vi "getCalibPoint.vi"(9 "y size":i32, 10 "pixel angel (y)":dbl[](array[numeric]), 11 "Momentum [MeV/C]":dbl[](array[numeric])) -> (0 "Array":dbl[][](array[numeric]), 1 "XY Graph 2":cluster{"X":dbl, "Y":dbl}[](graph), 2 "Reference Points":T1, 3 "output cluster":T1, 4 "XY Graph":cluster{"X":dbl, "Y":dbl}[](graph))   [LabVIEW 2011]
uses:
  <vilib>/vision/Calibration.llb/Calibration Reference Points.ctl
  <vilib>/Analysis/1siggen.llb/Ramp Pattern by Delta.vi
  <vilib>/Analysis/NI_AALBase.lvlib
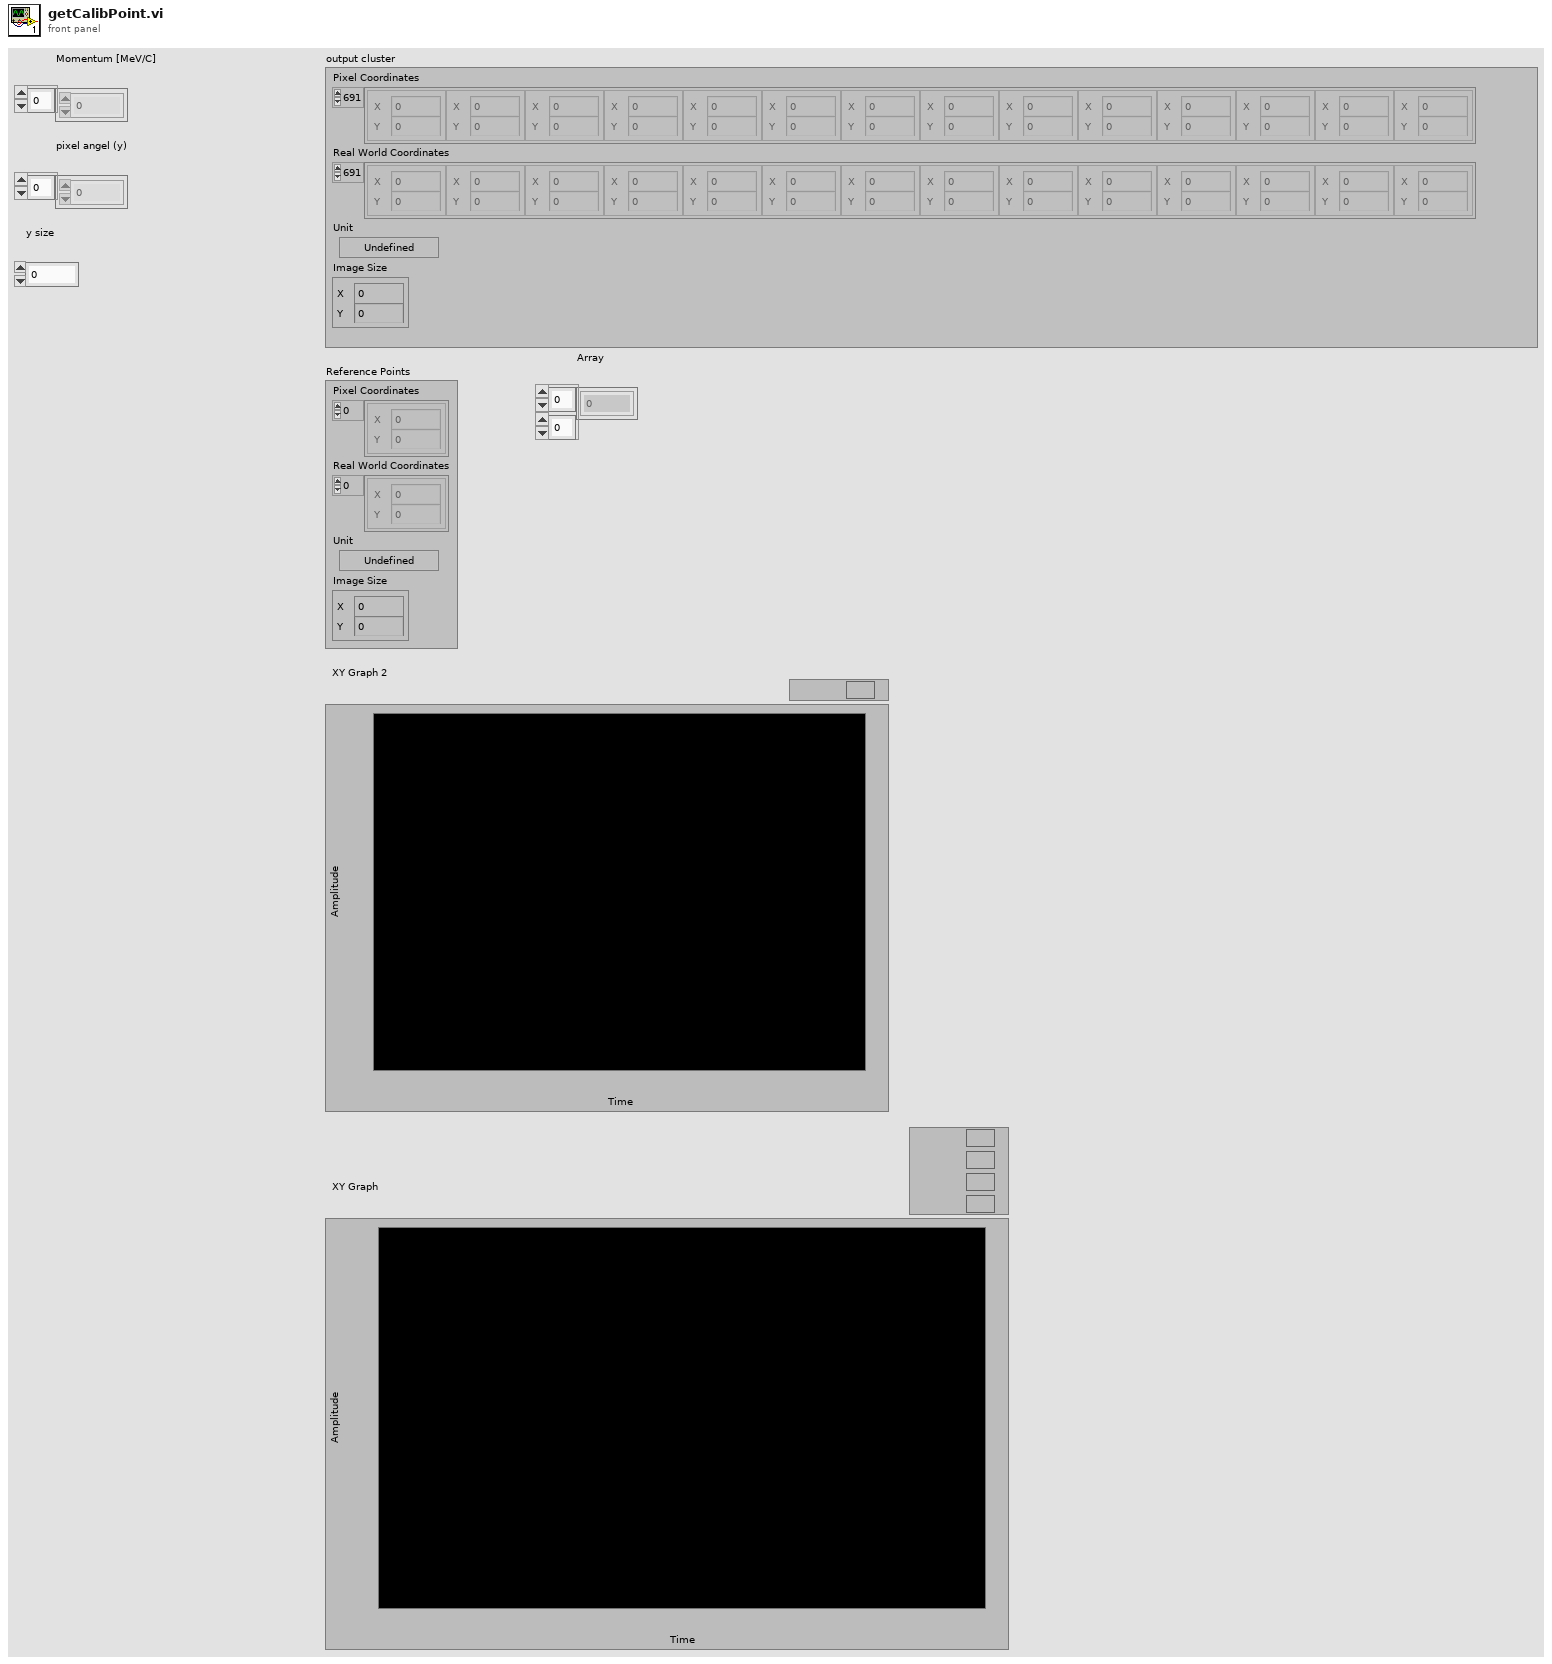
[diagram p1: front panel]
types:
  T1 = typedef "Calibration Reference Points.ctl" = cluster{"Pixel Coordinates":cluster{"X":dbl, "Y":dbl}[], "Real World Coordinates":cluster{"X":dbl, "Y":dbl}[], "Unit":T2, "Image Size":cluster{"X":u32, "Y":u32}}
  T2 = typedef "Image Unit" = enum32{"Undefined", "Angström", "Micrometer", "Millimeter", "Centimeter", "Meter", "Kilometer", "Microinch", "Inch", "Feet", "Nautical miles", "Standard miles", "Steps"}
  T3 = cluster{"Real Matrix Element":dbl, "Real Matrix Element":dbl}[]
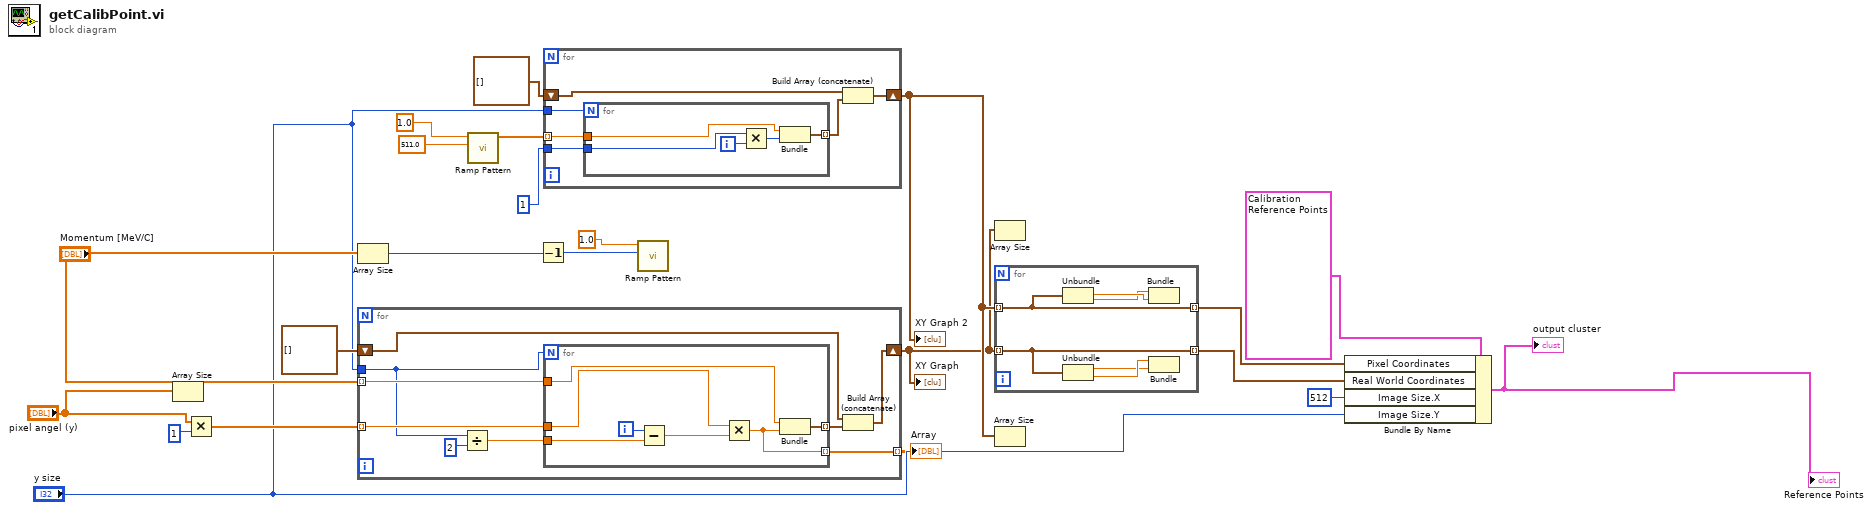
[diagram p0: block diagram]
diagram:
  n1 = Array Size(array="pixel angel (y)") -> ()  [unwired: 1 out]
  n2 = Multiply(x="pixel angel (y)", y=1) -> (x*y=w19:dbl[])
  n3 = Array Size(array="Momentum [MeV/C]") -> (size(s)=w10:i32)
  n4 = for {
    tunnel: "Momentum [MeV/C]" -> [w31] mode=indexing
    tunnel: "y size" -> [w26]
    shift-right: [w28] -> w20
    shift-left: cluster{dbl, dbl}[] [] -> [w29]
    tunnel: w19 -> [w27] mode=indexing
    tunnel: [w23] -> w1 mode=indexing
    n5 = Divide(x=w26, y=2) -> (x/y=w24:dbl)
    n6 = for {
      N: w26 -> [_]
      tunnel: w27 -> [w36]
      tunnel: w31 -> [w38]
      tunnel: [w37] -> w30 mode=indexing
      tunnel: w24 -> [w35]
      tunnel: [w32] -> w23 mode=indexing
      i -> [w33]
      n7 = Subtract(x=w33, y=w35) -> (x-y=w34:dbl)
      n8 = Multiply(x=w36, y=w34) -> (x*y=w32:dbl)
      n9 = Bundle(w38, w32) -> (w37:cluster{dbl, dbl})  [unwired: 1 in]
    }
    n10 = Build Array (concatenate)(w29, w30) -> (w28:cluster{dbl, dbl}[])
  }
  "XY Graph" <- w20
  "Array" <- w1
  n11 = call-poly <vilib>:"Ramp Pattern.vi"("end"=511.0, "delta"=1.0) -> ("Ramp Pattern"=w15:dbl[])  [unwired: 7 in, 2 out]
  n12 = Decrement(x=w10) -> (x-1=w11:i32)
  n13 = for {
    tunnel: w15 -> [w44] mode=indexing
    shift-right: [w42] -> w21
    shift-left: T3 [] -> [w41]
    tunnel: "y size" -> [w40]
    tunnel: 1 -> [w39]
    n14 = for {
      N: w40 -> [_]
      tunnel: w44 -> [w49]
      tunnel: [w48] -> w43 mode=indexing
      tunnel: w39 -> [w47]
      i -> [w45]
      n15 = Multiply(x=w47, y=w45) -> (x*y=w46:i32)
      n16 = Bundle(w49, w46) -> (w48:cluster{dbl, i32})  [unwired: 1 in]
    }
    n17 = Build Array (concatenate)(w41, w43) -> (w42:T3)
  }
  "XY Graph 2" <- w21
  n18 = call-poly <vilib>:"Ramp Pattern.vi"("end"=w11, "delta"=1.0) -> ()  [unwired: 7 in, 3 out]
  n19 = Array Size(array=w20) -> ()  [unwired: 1 out]
  n20 = for {
    tunnel: w21 -> [w50] mode=indexing
    tunnel: [w50] -> w7 mode=indexing
    tunnel: w20 -> [w51] mode=indexing
    tunnel: [w51] -> w8 mode=indexing
    n21 = Unbundle(w50) -> ("Real Matrix Element"=w55:dbl, "Real Matrix Element"=w54:dbl)
    n22 = Unbundle(w51) -> (w52:dbl, w53:dbl)
    n23 = Bundle("Real Matrix Element"=w54, "Real Matrix Element"=w55) -> ()  [unwired: 1 in, 1 out]
    n24 = Bundle(w53, w52) -> ()  [unwired: 1 in, 1 out]
  }
  n25 = Array Size(array=w21) -> ()  [unwired: 1 out]
  n26 = Bundle By Name(cluster=T1 {"Pixel Coordinates"=[{"X"=570.6379853095488, "Y"=340.45645330535154}, {"X"=647.5556818181818, "Y"=339.9465909090909}, {"X"=489.14118792599805, "Y"=340.794547224927}, {"X"=570.559915164369, "Y"=428.96182396606577}, {"X"=571.1038421599169, "Y"=251.64797507788163}, {"X"=719.6135802469136, "Y"=339.39012345679015}, {"X"=647.359212050985, "Y"=425.63731170336035}, {"X"=647.927355278093, "Y"=253.88081725312145}, {"X"=403.34514078110806, "Y"=341.1798365122616}, {"X"=489.36614173228344, "Y"=432.1003937007874}, {"X"=489.63300970873786, "Y"=249.25242718446603}, {"X"=570.873775843308, "Y"=516.2143634385201}, {"X"=571.809968847352, "Y"=163.4288681204569}, {"X"=786.8324396782842, "Y"=338.73458445040217}, {"X"=719.1072319201995, "Y"=422.27431421446386}, {"X"=719.8995098039215, "Y"=256.234068627451}, {"X"=647.1241134751773, "Y"=510.1111111111111}, {"X"=648.2274774774775, "Y"=168.53603603603602}, {"X"=313.9448751076658, "Y"=341.3255813953488}, {"X"=403.84508348794066, "Y"=434.9007421150278}, {"X"=404.0036199095023, "Y"=247.020814479638}, {"X"=490.1742654508612, "Y"=521.9088145896657}, {"X"=490.8612997090204, "Y"=158.447138700291}, {"X"=571.4618834080718, "Y"=601.1838565022422}, {"X"=572.9046121593292, "Y"=76.90041928721175}, {"X"=849.2731277533039, "Y"=338.05286343612335}, {"X"=786.2282608695652, "Y"=418.85733695652175}, {"X"=787.0280748663101, "Y"=258.451871657754}, {"X"=718.5839694656488, "Y"=504.147582697201}, {"X"=720.0232843137255, "Y"=173.4950980392157}, {"X"=647.0180940892642, "Y"=592.6731001206273}, {"X"=648.7929465301479, "Y"=84.46416382252559}, {"X"=221.77860082304528, "Y"=341.1670781893004}, {"X"=314.82819383259914, "Y"=437.3339207048458}, {"X"=314.7304721030043, "Y"=244.76223175965666}, {"X"=405.3212927756654, "Y"=527.143536121673}, {"X"=405.59471766848816, "Y"=153.63934426229508}, {"X"=491.61099585062243, "Y"=609.1804979253112}, {"X"=492.59488692232054, "Y"=69.41297935103245}, {"X"=907.184126984127, "Y"=337.3492063492063}, {"X"=848.5985401459855, "Y"=415.5036496350365}, {"X"=849.5179340028694, "Y"=260.5337159253946}, {"X"=785.3477051460361, "Y"=497.970792767733}, {"X"=787.0389784946236, "Y"=178.5}, {"X"=717.9280104712042, "Y"=584.0955497382199}, {"X"=719.9565756823821, "Y"=92.06699751861042}, {"X"=647.0678391959799, "Y"=672.3969849246231}, {"X"=128.00558659217876, "Y"=340.95211492418196}, {"X"=223.03713080168777, "Y"=439.37215189873416}, {"X"=222.6743232157506, "Y"=242.66119770303527}, {"X"=317.0428954423592, "Y"=531.9240393208222}, {"X"=316.9982593559617, "Y"=149.05657093124455}, {"X"=407.8424124513619, "Y"=616.7752918287938}, {"X"=408.35483870967744, "Y"=62.259907834101384}, {"X"=960.7057823129252, "Y"=336.69727891156464}, {"X"=907.3485086342229, "Y"=262.6734693877551}, {"X"=906.4731012658228, "Y"=412.1107594936709}, {"X"=847.4038748137109, "Y"=491.89120715350225}, {"X"=849.2749638205499, "Y"=183.3589001447178}, {"X"=784.1076487252125, "Y"=575.3881019830028}, {"X"=786.4362416107383, "Y"=99.71677852348994}, {"X"=717.0723860589812, "Y"=661.4302949061662}, {"X"=34.00241351568785, "Y"=340.5036202735318}, {"X"=129.57247557003257, "Y"=440.9112377850163}, {"X"=128.98718975180145, "Y"=240.6781425140112}, {"X"=226.0763948497854, "Y"=535.91330472103}, {"X"=225.50957535387178, "Y"=144.7993338884263}, {"X"=320.5830258302583, "Y"=623.5516605166051}, {"X"=320.6681338028169, "Y"=55.44718309859155}, {"X"=959.902229845626, "Y"=408.7667238421955}, {"X"=961.0357142857143, "Y"=264.4761904761905}, {"X"=906.8826291079812, "Y"=188.11111111111111}, {"X"=905.0571895424837, "Y"=485.84313725490193}, {"X"=845.760606060606, "Y"=566.7060606060606}, {"X"=848.4970674486804, "Y"=107.16275659824046}, {"X"=782.7893217893218, "Y"=650.4559884559884}, {"X"=785.8817802503477, "Y"=23.17385257301808}, {"X"=35.88134206219313, "Y"=441.8216039279869}, {"X"=35.05444355484388, "Y"=238.72858286629304}, {"X"=133.46192052980132, "Y"=538.9850993377484}, {"X"=132.46532258064516, "Y"=141.14032258064515}, {"X"=230.79331574318383, "Y"=629.3078276165347}, {"X"=230.16807432432432, "Y"=49.3902027027027}, {"X"=958.3894736842105, "Y"=479.9719298245614}, {"X"=960.3236301369863, "Y"=192.6318493150685}, {"X"=905.9124203821656, "Y"=114.5859872611465}, {"X"=903.1179401993355, "Y"=558.3671096345515}, {"X"=843.9289099526067, "Y"=639.6808846761453}, {"X"=847.2578710644677, "Y"=32.788605697151425}, {"X"=40.43729372937294, "Y"=541.0767326732673}, {"X"=39.07723250201126, "Y"=138.17940466613032}, {"X"=139.56319862424763, "Y"=633.9475494411006}, {"X"=138.17063166529942, "Y"=44.12059064807219}, {"X"=956.1873905429072, "Y"=550.2416812609457}, {"X"=959.1889081455806, "Y"=121.45580589254766}, {"X"=904.3951612903226, "Y"=42.28709677419355}, {"X"=900.7631133671742, "Y"=629.0304568527919}, {"X"=47.85025817555938, "Y"=637.2874354561102}, {"X"=45.69761709120789, "Y"=39.833196384552174}, {"X"=953.6286231884058, "Y"=618.5615942028985}, {"X"=957.3913043478261, "Y"=51.740869565217395}], "Real World Coordinates"=[{"X"=60.0, "Y"=30.0}, {"X"=70.0, "Y"=30.0}, {"X"=50.0, "Y"=30.0}, {"X"=60.0, "Y"=40.0}, {"X"=60.0, "Y"=20.0}, {"X"=80.0, "Y"=30.0}, {"X"=70.0, "Y"=40.0}, {"X"=70.0, "Y"=20.0}, {"X"=40.0, "Y"=30.0}, {"X"=50.0, "Y"=40.0}, {"X"=50.0, "Y"=20.0}, {"X"=60.0, "Y"=50.0}, {"X"=60.0, "Y"=10.0}, {"X"=90.0, "Y"=30.0}, {"X"=80.0, "Y"=40.0}, {"X"=80.0, "Y"=20.0}, {"X"=70.0, "Y"=50.0}, {"X"=70.0, "Y"=10.0}, {"X"=30.0, "Y"=30.0}, {"X"=40.0, "Y"=40.0}, {"X"=40.0, "Y"=20.0}, {"X"=50.0, "Y"=50.0}, {"X"=50.0, "Y"=10.0}, {"X"=60.0, "Y"=60.0}, {"X"=60.0, "Y"=0.0}, {"X"=100.0, "Y"=30.0}, {"X"=90.0, "Y"=40.0}, {"X"=90.0, "Y"=20.0}, {"X"=80.0, "Y"=50.0}, {"X"=80.0, "Y"=10.0}, {"X"=70.0, "Y"=60.0}, {"X"=70.0, "Y"=0.0}, {"X"=20.0, "Y"=30.0}, {"X"=30.0, "Y"=40.0}, {"X"=30.0, "Y"=20.0}, {"X"=40.0, "Y"=50.0}, {"X"=40.0, "Y"=10.0}, {"X"=50.0, "Y"=60.0}, {"X"=50.0, "Y"=0.0}, {"X"=110.0, "Y"=30.0}, {"X"=100.0, "Y"=40.0}, {"X"=100.0, "Y"=20.0}, {"X"=90.0, "Y"=50.0}, {"X"=90.0, "Y"=10.0}, {"X"=80.0, "Y"=60.0}, {"X"=80.0, "Y"=0.0}, {"X"=70.0, "Y"=70.0}, {"X"=10.0, "Y"=30.0}, {"X"=20.0, "Y"=40.0}, {"X"=20.0, "Y"=20.0}, {"X"=30.0, "Y"=50.0}, {"X"=30.0, "Y"=10.0}, {"X"=40.0, "Y"=60.0}, {"X"=40.0, "Y"=0.0}, {"X"=120.0, "Y"=30.0}, {"X"=110.0, "Y"=20.0}, {"X"=110.0, "Y"=40.0}, {"X"=100.0, "Y"=50.0}, {"X"=100.0, "Y"=10.0}, {"X"=90.0, "Y"=60.0}, {"X"=90.0, "Y"=0.0}, {"X"=80.0, "Y"=70.0}, {"X"=0.0, "Y"=30.0}, {"X"=10.0, "Y"=40.0}, {"X"=10.0, "Y"=20.0}, {"X"=20.0, "Y"=50.0}, {"X"=20.0, "Y"=10.0}, {"X"=30.0, "Y"=60.0}, {"X"=30.0, "Y"=0.0}, {"X"=120.0, "Y"=40.0}, {"X"=120.0, "Y"=20.0}, {"X"=110.0, "Y"=10.0}, {"X"=110.0, "Y"=50.0}, {"X"=100.0, "Y"=60.0}, {"X"=100.0, "Y"=0.0}, {"X"=90.0, "Y"=70.0}, {"X"=90.0, "Y"=-10.0}, {"X"=0.0, "Y"=40.0}, {"X"=0.0, "Y"=20.0}, {"X"=10.0, "Y"=50.0}, {"X"=10.0, "Y"=10.0}, {"X"=20.0, "Y"=60.0}, {"X"=20.0, "Y"=0.0}, {"X"=120.0, "Y"=50.0}, {"X"=120.0, "Y"=10.0}, {"X"=110.0, "Y"=0.0}, {"X"=110.0, "Y"=60.0}, {"X"=100.0, "Y"=70.0}, {"X"=100.0, "Y"=-10.0}, {"X"=0.0, "Y"=50.0}, {"X"=0.0, "Y"=10.0}, {"X"=10.0, "Y"=60.0}, {"X"=10.0, "Y"=0.0}, {"X"=120.0, "Y"=60.0}, {"X"=120.0, "Y"=0.0}, {"X"=110.0, "Y"=-10.0}, {"X"=110.0, "Y"=70.0}, {"X"=0.0, "Y"=60.0}, {"X"=0.0, "Y"=0.0}, {"X"=120.0, "Y"=70.0}, {"X"=120.0, "Y"=-10.0}], "Unit"=enum."Millimeter", "Image Size"={"X"=1000, "Y"=700}} ("Reference Points"), "Pixel Coordinates"=w7, "Real World Coordinates"=w8, "Image Size.X"=u32 512, "Image Size.Y"="y size") -> (→"output cluster" →"Reference Points":T1)
